vi "Remove Package from SystemLink Feed (By Name).vi"(0 "SystemLink repo in":T1, 5 "feed name in":string, 7 "package name":string, 9 "package version":string, 11 "error in (no error)":errorcluster, 12 "timeout (ms) (10000)":u32=10000) -> (4 "SystemLink repo out":T1, 6 "feed name out":string, 10 "timed out?":bool, 15 "error out":errorcluster)   [LabVIEW 2017, in "SystemLink_Repo_API.lvlib"]
doc: "Removes the package from a SystemLink feed. Specify the package by its name and version.\n\nNote: If the removed package is no longer referenced by any other feeds, the package will be automatically deleted from the SystemLink package repository.\n\nError Handling:\nReturns an error if the specified package or feed does not exist in the SystemLink repository."
uses:
  SystemLink_Repo_API.lvlib
  <vilib>/httpClient/ClientHandle.ctl
  <vilib>/httpClient/LabVIEWHTTPClient.lvlib
  _support/systemlink repo.ctl
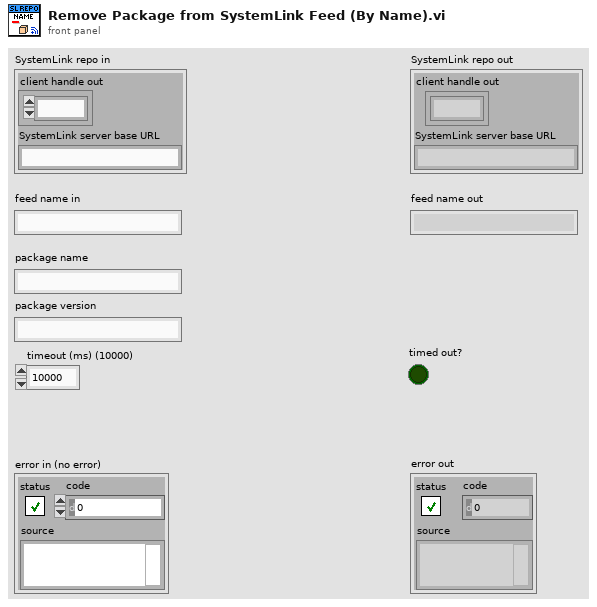
[diagram p1: front panel]
types:
  T1 = typedef "SystemLink_Repo_API.lvlib/systemlink repo.ctl" = cluster{"client handle out":T2, "SystemLink server base URL":string}
  T2 = typedef "LabVIEWHTTPClient.lvlib/ClientHandle.ctl" = refnum<k1>
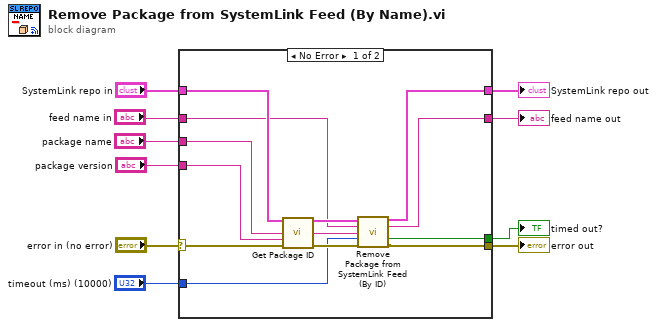
[diagram p0: block diagram]
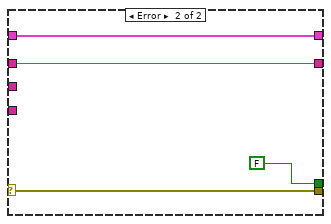
[diagram p2: hidden frame]
diagram:
  n1 = case shown="No Error" "error in (no error)" {
    selector: "error in (no error)" -> [w16 w27]
    tunnel: "SystemLink repo in" -> [w23 w26]
    tunnel: [w13 w27] -> w8
    tunnel: [w12 w26] -> w7
    tunnel: "feed name in" -> [w18 w24]
    tunnel: "package name" -> [w20 _]
    tunnel: "timeout (ms) (10000)" -> [w15 _]
    tunnel: [w14 FALSE ("timed out?")] -> w3
    tunnel: "package version" -> [w21 _]
    tunnel: [w11 w24] -> w1
    frame No Error {
      n2 = call "Get Package ID.vi"("SystemLink repo in"=w23, "package name"=w20, "package version"=w21, "error in (no error)"=w16) -> ("SystemLink repo out"=w22:T1, "package ID"=w19:string, "error out"=w17:errorcluster)  [unwired: 9 in]
      n3 = call "Remove Package from SystemLink Feed (By ID).vi"("SystemLink repo in"=w22, "feed name in"=w18, "package ID"=w19, "timeout (ms) (10000)"=w15, "error in (no error)"=w17) -> ("SystemLink repo out"=w12:T1, "feed name out"=w11:string, "timed out?"=w14:bool, "error out"=w13:errorcluster)  [unwired: 7 in]
    }
    frame Error {
    }
  }
  "error out" <- w8
  "SystemLink repo out" <- w7
  "feed name out" <- w1
  "timed out?" <- w3
